vi "HFRR ADV v01.vi"() -> ()   [LabVIEW 2025] (continued)
            n2592 = Concatenate Strings(w3366, ".duf" ("Substring")) -> (w3363:string)
            n2593 = String To Path(string=w3363) -> (path=w3361:path)
            n2594 = call <vilib>:"Read Characters From File.vi"("file path (dialog if empty)"=w3361, "start of read offset (chars.:0)"=60 ("start of read offset (chars.: 0)")) -> ("character string"=→"String Control 4":string)  [unwired: 4 in, 3 out]
          }
        }
        n2595 = case shown="True" "OPEN 3" {
          frame False {
          }
          frame True {
            (unwired) 0  # existing file
            w3387 = "Choose a datalog file to open"  # prompt
            n2596 = local write "OPEN 3"(FALSE ("OPEN 1")) -> ()
            n2597 = String To Path(string="C:\\LAB-IQ\\Data\\") -> (path=w3372:path)
            n2598 = File Dialog(6:"*.dgf" ("pattern"), 7:w3387, 11:w3372) -> (0:w3370:errorcluster, 3:w3378:path)  [unwired: 4 in, 2 out]
            n2599 = Unbundle(w3370) -> ()  [unwired: 3 out]
            n2600 = Strip Path(path=w3378) -> (name=w3376:string)  [unwired: 1 out]
            n2601 = Path To String(path=w3378) -> (string=w3373:string)
            "string1 3" <- w3373
            n2602 = Match Pattern(string=w3376, regular expression=".dgf") -> (before substring=→"String Control 5":string)  [unwired: 1 in, 3 out]
            n2603 = Match Pattern(string=w3373, regular expression=".dgf" ("substring (\"\")")) -> (before substring=w3383:string)  [unwired: 1 in, 3 out]
            n2604 = Concatenate Strings(w3383, ".duf" ("Substring")) -> (w3380:string)
            n2605 = String To Path(string=w3380) -> (path=w3384:path)
            n2606 = call <vilib>:"Read Characters From File.vi"("file path (dialog if empty)"=w3384, "start of read offset (chars.:0)"=60 ("start of read offset (chars.: 0)")) -> ("character string"=→"String Control 6":string)  [unwired: 4 in, 3 out]
          }
        }
        n2607 = case shown="True" "OPEN 4" {
          frame False {
          }
          frame True {
            (unwired) 0  # existing file
            w3405 = "Choose a datalog file to open"  # prompt
            n2608 = local write "OPEN 4"(FALSE ("OPEN 1")) -> ()
            n2609 = String To Path(string="C:\\LAB-IQ\\Data\\") -> (path=w3390:path)
            n2610 = File Dialog(6:"*.dgf" ("pattern"), 7:w3405, 11:w3390) -> (0:w3388:errorcluster, 3:w3396:path)  [unwired: 4 in, 2 out]
            n2611 = Unbundle(w3388) -> ()  [unwired: 3 out]
            n2612 = Strip Path(path=w3396) -> (name=w3394:string)  [unwired: 1 out]
            n2613 = Path To String(path=w3396) -> (string=w3391:string)
            "string1 4" <- w3391
            n2614 = Match Pattern(string=w3394, regular expression=".dgf") -> (before substring=→"String Control 7":string)  [unwired: 1 in, 3 out]
            n2615 = Match Pattern(string=w3391, regular expression=".dgf" ("substring (\"\")")) -> (before substring=w3401:string)  [unwired: 1 in, 3 out]
            n2616 = Concatenate Strings(w3401, ".duf" ("Substring")) -> (w3398:string)
            n2617 = String To Path(string=w3398) -> (path=w3402:path)
            n2618 = call <vilib>:"Read Characters From File.vi"("file path (dialog if empty)"=w3402, "start of read offset (chars.:0)"=60 ("start of read offset (chars.: 0)")) -> ("character string"=→"String Control 8":string)  [unwired: 4 in, 3 out]
          }
        }
      }
      frame "About" {
        # "Elapsed time\ncof\nstroke\nmean pos\nTemp\nHumidity"
        n2619 = disable-structure shown="Disabled" {
          frame Disabled {
            n2620 = case shown="True" "Export" {
              frame False {
              }
              frame True {
                w3427 = "                                      " ("string")
                w3429 = "\r"
                (unwired) i16 6 ("width (-)")
                w3506 = "\r"
                w3438 = "\r"
                n2621 = local write "Export"(FALSE ("Export")) -> ()
                n2622 = local read "String 29"() -> (w3475:string)
                n2623 = local read "String 34"() -> (w3463:string)
                n2624 = local read "String 35"() -> (w3458:string)
                n2625 = local read "String 37"() -> (w3454:string)
                n2626 = local read "String 36"() -> (w3451:string)
                n2627 = local read "String 38"() -> (w3448:string)
                n2628 = local read "String 39"() -> (w3445:string)
                n2629 = Match Pattern(string=w3475, regular expression=".dwm") -> (before substring=w3471:string)  [unwired: 1 in, 3 out]
                "before substring" <- w3471
                n2630 = local read "S 38"() -> (w3466:string)
                n2631 = local read "S 39"() -> (w3459:string)
                n2632 = local read "Temperature before test 2"() -> (w3495:dbl)
                n2633 = local read "Temperature after test 2"() -> (w3500:dbl)
                n2634 = local read "Humidity before test 2"() -> (w3481:dbl)
                n2635 = local read "Humidity after test 2"() -> (w3496:dbl)
                n2636 = local read "MWSD 2"() -> (w3492:dbl)
                n2637 = local read "WS1.4 2"() -> (w3508:dbl)
                n2638 = local read "HCF 2"() -> (w3504:dbl)
                n2639 = local read "AVP 2"() -> (w3493:dbl)
                n2640 = Concatenate Strings("1," ("string"), w3466) -> (w3465:string)
                n2641 = Concatenate Strings("2," ("string"), w3463) -> (w3462:string)
                n2642 = Concatenate Strings("3," ("string"), w3459) -> (w3461:string)
                n2643 = Concatenate Strings("4," ("string"), w3458) -> (w3457:string)
                n2644 = Concatenate Strings("5," ("string"), w3454) -> (w3455:string)
                n2645 = Concatenate Strings("6," ("string"), w3451) -> (w3452:string)
                n2646 = Concatenate Strings("7," ("string"), w3448) -> (w3449:string)
                n2647 = Concatenate Strings("8," ("string"), w3445) -> (w3446:string)
                n2648 = local read "Sample ID"() -> (w3513:string)
                n2649 = case shown="\"xlx\"" "Select File Type" {
                  tunnel: w3471 -> [w3516 w3518 w3520]
                  tunnel: [w3514 w3519 w3521] -> w3470
                  frame "xlx" {
                    n2650 = Concatenate Strings(w3516, ".xls" ("string")) -> (w3514:string)
                  }
                  frame "csv" {
                    n2651 = Concatenate Strings(w3518, ".csv" ("string")) -> (w3519:string)
                  }
                  frame "txt" {
                    n2652 = Concatenate Strings(w3520, ".txt" ("string")) -> (w3521:string)
                  }
                }
                n2653 = local read "Test Date"() -> (w3512:string)
                n2654 = local read "String 45"() -> (w3426:string)
                n2655 = local read "String 31"() -> (w3511:string)
                n2656 = local read "String 32"() -> (w3510:string)
                n2657 = local read "TITTLE"() -> (w3434:string)
                n2658 = Number To Fractional String(number=w3481, width (-)=i16 6, precision (6)=i16 2) -> (F-format string=w3480:string)  [unwired: 1 in]
                n2659 = Number To Fractional String(number=w3495, width (-)=i16 6, precision (6)=i16 2) -> (F-format string=w3501:string)  [unwired: 1 in]
                n2660 = Number To Fractional String(number=w3496, width (-)=i16 6, precision (6)=i16 2) -> (F-format string=w3494:string)  [unwired: 1 in]
                n2661 = Number To Fractional String(number=w3500, width (-)=i16 6, precision (6)=i16 2) -> (F-format string=w3499:string)  [unwired: 1 in]
                n2662 = Number To Fractional String(number=w3492, width (-)=i16 6, precision (6)=i16 2) -> (F-format string=w3490:string)  [unwired: 1 in]
                n2663 = Number To Fractional String(number=w3493, width (-)=i16 6, precision (6)=i16 2) -> (F-format string=w3491:string)  [unwired: 1 in]
                n2664 = Number To Fractional String(number=w3504, width (-)=i16 6, precision (6)=i16 2) -> (F-format string=w3505:string)  [unwired: 1 in]
                n2665 = Number To Fractional String(number=w3508, precision (6)=i16 2) -> (F-format string=w3509:string)  [unwired: 2 in]
                n2666 = local read "s.NO"() -> (w3428:string)
                n2667 = Concatenate Strings("=" ("string"), w3434) -> (w3433:string)
                n2668 = Concatenate Strings("S.No," ("string"), "                                       Parameters" ("string")) -> (w3439:string)
                n2669 = Concatenate Strings(w3506, w3465, w3480, w3506, w3462, w3501, w3506, w3461, w3494, w3506, w3457, w3499, w3506, w3455, w3490, w3506, w3452, w3491, w3506, w3449, w3505, w3506, w3446, w3509) -> (w3468:string)
                n2670 = Concatenate Strings(w3438, "," ("string"), w3426, w3428, w3427, w3510, w3513, w3427, w3511, w3512, w3438) -> (w3436:string)
                n2671 = local read "Tested by"() -> (w3442:string)
                n2672 = local read "String 33"() -> (w3443:string)
                n2673 = Concatenate Strings("," ("string"), "                                                                             " ("string")) -> (w3431:string)
                n2674 = Concatenate Strings(w3433, w3429, w3436, w3429, w3439, w3468, w3429, w3431, w3443, w3442) -> (→"export":string)
                n2675 = String To Path(string=w3470) -> (path=w3477:path)
                n2676 = local read "export"() -> (w3472:string)
                n2677 = call <vilib>:"Write Characters To File.vi"("append to file? (new file:F)"=FALSE, "character string"=w3472, "file path (dialog if empty)"=w3477) -> ()  [unwired: 2 in, 1 out]
              }
            }
          }
          frame Enabled {
          }
        }
        n2678 = case shown="True" "OK Button 17" {
          frame False {
          }
          frame True {
            (unwired) 0  # existing file
            w3730 = "Choose a datalog file to open"  # prompt
            n2679 = local write "OK Button 17"(FALSE ("OK Button 17")) -> ()
            n2680 = local read "String"() -> (w3725:string)
            n2681 = String To Path(string=w3725) -> (path=w3726:path)
            n2682 = File Dialog(6:"*.duf" ("pattern"), 7:w3730, 11:w3726) -> (0:w3717:errorcluster, 3:w3736:path)  [unwired: 4 in, 2 out]
            n2683 = Unbundle(w3717) -> ()  [unwired: 3 out]
            n2684 = Open/Create/Replace File "Open File"(file path (use dialog)=w3736) -> (refnum out=w3728:refnum<file>)  [unwired: 5 in, 2 out]
            n2685 = Strip Path(path=w3736) -> (name=w3734:string)  [unwired: 1 out]
            n2686 = Path To String(path=w3736) -> (string=w3719:string)
            n2687 = while {
              tunnel: w3728 -> [w3740]
              i -> [w3737]
              stop <- w3738 continue-if-true
              (unwired) TRUE ("line mode (F)")
              n2688 = Read from Text File "Read File"(file (use dialog)=w3740) -> (text=w3739:string)  [unwired: 3 in, 3 out]
              n2689 = local write "Numeric 16"(w3737) -> ()
              n2690 = String Length(string=w3739) -> (length=w3742:i32)
              n2691 = Greater?(x=w3742, y=1) -> (0:w3738:bool)
            }
            n2692 = local write "String 29"(w3719) -> ()
            n2693 = Search and Replace String(input string=w3719, search string=".duf", replace string=".dgf" ("replace string (\"\")")) -> (result string=→"String Indicator 4":string)  [unwired: 5 in, 3 out]
            n2694 = Match Pattern(string=w3734, regular expression=".dwm") -> (before substring=w3718:string)  [unwired: 1 in, 3 out]
            "String Indicator" <- w3718
            n2695 = Match Pattern(string=w3719, regular expression=".dwm" ("substring (\"\")")) -> (before substring=w3720:string)  [unwired: 1 in, 3 out]
            "String Indicator 3" <- w3720
            n2696 = local write "TITTLE 2"(w3718) -> ()
            n2697 = String To Path(string=w3720) -> (path=w3727:path)
            "path" <- w3727
            n2698 = call <vilib>:"Read Characters From File.vi"("file path (dialog if empty)"=w3727, "start of read offset (chars.:0)"=60 ("start of read offset (chars.: 0)")) -> ("character string"=→"String Indicator 2":string)  [unwired: 4 in, 3 out]
          }
        }
        n2699 = call <vilib>:"Query Available Printers.vi"() -> ("system configured printers"=w3419:string[])  [unwired: 9 in, 2 out]
        "System Configured Printers 2" <- w3419
        n2700 = local read "OK Button 16"() -> (w3416:bool)
        n2701 = case shown="True" "OK Button 16" {
          frame False {
          }
          frame True {
            n2702 = stacked-sequence {
              frame #0 {
                n2703 = local read "Numeric 16"() -> (w3744:i32)
                n2704 = local write "Numeric 10"(w3744) -> ()
              }
              frame #1 {
                n2705 = local read "S.NO"() -> (→"s.NO":string)
                n2706 = local read "String 29"() -> (w3748:string)
                n2707 = String To Path(string=w3748) -> (path=w3747:path)
                n2708 = Open/Create/Replace File "Open File"(file path (use dialog)=w3747) -> (refnum out=w3749:refnum<file>)  [unwired: 5 in, 2 out]
                n2709 = for {
                  N: 16 -> [_]
                  tunnel: w3749 -> [w3756]
                  i -> [w3752]
                  (unwired) TRUE ("line mode (F)")
                  n2710 = Read from Text File "Read File"(file (use dialog)=w3756) -> (text=w3750:string)  [unwired: 3 in, 3 out]
                  n2711 = Match Pattern(string=w3750, regular expression="(") -> (after substring=w3755:string)  [unwired: 1 in, 3 out]
                  n2712 = Match Pattern(string=w3755, regular expression=")") -> (before substring=w3751:string)  [unwired: 1 in, 3 out]
                  n2713 = case shown="1" w3752 {
                    tunnel: w3751 -> [w3757 w3758 _ _ w3759 w3760 w3761 w3763 w3765 w3767 w3769 w3771 w3773 w3775 _]
                    tunnel: w3750 -> [_ _ _ _ _ _ _ _ _ _ _ _ _ _ _]
                    frame 0 {
                      "TITTLE" <- w3757
                    }
                    frame 1 {
                      "Sample ID" <- w3758
                    }
                    frame 2 {
                    }
                    frame 3 {
                    }
                    frame 4 {
                      "Test Date" <- w3759
                    }
                    frame 5 {
                      "Tested by" <- w3760
                    }
                    frame 6 {
                      n2714 = Fract/Exp String To Number(string=w3761) -> (number=→"Humidity before test 2":dbl)  [unwired: 3 in, 1 out]
                    }
                    frame 7 {
                      n2715 = Fract/Exp String To Number(string=w3763) -> (number=→"Temperature before test 2":dbl)  [unwired: 3 in, 1 out]
                    }
                    frame 8 {
                      n2716 = Fract/Exp String To Number(string=w3765) -> (number=→"Humidity after test 2":dbl)  [unwired: 3 in, 1 out]
                    }
                    frame 9 {
                      n2717 = Fract/Exp String To Number(string=w3767) -> (number=→"Temperature after test 2":dbl)  [unwired: 3 in, 1 out]
                    }
                    frame 10 {
                      n2718 = Fract/Exp String To Number(string=w3769) -> (number=→"MWSD 2":dbl)  [unwired: 3 in, 1 out]
                    }
                    frame 11 {
                      n2719 = Fract/Exp String To Number(string=w3771) -> (number=→"AVP 2":dbl)  [unwired: 3 in, 1 out]
                    }
                    frame 12 {
                      n2720 = Fract/Exp String To Number(string=w3773) -> (number=→"HCF 2":dbl)  [unwired: 3 in, 1 out]
                    }
                    frame 13 {
                      n2721 = Fract/Exp String To Number(string=w3775) -> (number=→"WS1.4 2":dbl)  [unwired: 3 in, 1 out]
                    }
                    frame 14, Default {
                    }
                  }
                }
              }
              frame #2 {
              }
            }
            n2722 = local write "OK Button 16"(FALSE ("OK Button 13")) -> ()
          }
        }
        n2723 = Index Array(array=w3419, index="Select Printer 3") -> (element=w3421:string)
        "Selected Printer" <- w3421
        n2724 = case shown="True" w3416 {
          frame False {
          }
          frame True {
            n2725 = flat-sequence {
              frame #0 {
              }
              frame #1 {
                n2726 = Wait (ms)(milliseconds to wait=u32 100) -> ()  [unwired: 1 out]
              }
              frame #2 {
                n2727 = local write "OK Button 16"(FALSE ("Print 3")) -> ()
              }
            }
          }
        }
        n2728 = case shown="True" "Print" {
          tunnel: w3421 -> [_ w3713]
          frame False {
          }
          frame True {
            (unwired) i16 6 ("width (-)")
            (unwired) "TESTED BY : "
            (unwired) "TESTED DATE :"
            (unwired) "SAMPLE ID : "
            (unwired) "SAMPLE DESIGN : "
            w3671 = "\r"
            w3688 = "\r"
            # "add image"
            n2729 = local read "Sample ID"() -> (w3661:string)
            n2730 = local read "Tested by"() -> (w3664:string)
            n2731 = local read "String 34"() -> (w3651:string)
            n2732 = local read "String 45"() -> (w3631:string)
            n2733 = local read "String 35"() -> (w3646:string)
            n2734 = local read "String 37"() -> (w3644:string)
            n2735 = local read "String 32"() -> (w3666:string)
            n2736 = local read "String 36"() -> (w3641:string)
            n2737 = local read "String 31"() -> (w3665:string)
            n2738 = local read "Test Date"() -> (w3662:string)
            n2739 = local read "String 33"() -> (w3667:string)
            n2740 = local read "String 38"() -> (w3637:string)
            n2741 = local read "String 39"() -> (w3634:string)
            n2742 = local write "Print"(FALSE ("Print FF")) -> ()
            n2743 = local read "S 39"() -> (w3649:string)
            n2744 = local read "S 38"() -> (w3656:string)
            n2745 = local read "Temperature before test 2"() -> (w3687:dbl)
            n2746 = local read "Temperature after test 2"() -> (w3677:dbl)
            n2747 = local read "Humidity before test 2"() -> (w3702:dbl)
            n2748 = local read "Humidity after test 2"() -> (w3686:dbl)
            n2749 = local read "MWSD 2"() -> (w3691:dbl)
            n2750 = local read "WS1.4 2"() -> (w3669:dbl)
            n2751 = Concatenate Strings("2)" ("string"), w3651) -> (w3652:string)
            n2752 = Concatenate Strings("3)" ("string"), w3649) -> (w3650:string)
            n2753 = Concatenate Strings("1)" ("string"), w3656) -> (w3655:string)
            n2754 = Concatenate Strings("4)" ("string"), w3646) -> (w3647:string)
            n2755 = Concatenate Strings("5)" ("string"), w3644) -> (w3643:string)
            n2756 = Concatenate Strings("6)" ("string"), w3641) -> (w3640:string)
            n2757 = Concatenate Strings("7)" ("string"), w3637) -> (w3638:string)
            n2758 = Concatenate Strings("8)" ("string"), w3634) -> (w3635:string)
            n2759 = local read "HCF 2"() -> (w3673:dbl)
            n2760 = local read "AVP 2"() -> (w3690:dbl)
            n2761 = local read "s.NO"() -> (w3632:string)
            n2762 = call <vilib>:"New Report.vi"("report type"=enum16{"Standard Report", "HTML"}."Standard Report") -> ("report out"=w3711:refnum<class "NI_report.lvclass">, "error out"=w3710:errorcluster)  [unwired: 13 in]
            n2763 = local read "TITTLE"() -> (w3663:string)
            n2764 = Concatenate Strings(w3688, w3631, w3632, w3688, w3666, w3661, w3688, w3665, w3662, w3688, w3667, w3664, w3688) -> (w3681:string)
            "test by" <- w3681
            n2765 = Number To Fractional String(number=w3687, width (-)=i16 6, precision (6)=i16 2) -> (F-format string=w3676:string)  [unwired: 1 in]
            n2766 = Number To Fractional String(number=w3686, width (-)=i16 6, precision (6)=i16 2) -> (F-format string=w3689:string)  [unwired: 1 in]
            n2767 = Number To Fractional String(number=w3702, width (-)=i16 6, precision (6)=i16 2) -> (F-format string=w3707:string)  [unwired: 1 in]
            n2768 = Number To Fractional String(number=w3691, width (-)=i16 6, precision (6)=i16 2) -> (F-format string=w3693:string)  [unwired: 1 in]
            n2769 = Number To Fractional String(number=w3677, width (-)=i16 6, precision (6)=i16 2) -> (F-format string=w3678:string)  [unwired: 1 in]
            n2770 = Number To Fractional String(number=w3690, width (-)=i16 6, precision (6)=i16 2) -> (F-format string=w3692:string)  [unwired: 1 in]
            n2771 = Number To Fractional String(number=w3673, width (-)=i16 6, precision (6)=i16 2) -> (F-format string=w3672:string)  [unwired: 1 in]
            n2772 = Number To Fractional String(number=w3669, precision (6)=i16 2) -> (F-format string=w3668:string)  [unwired: 2 in]
            n2773 = call-dynamic "Set Report Header Text.vi"("report in"=w3711, "center header text"=w3663, "error in (no error)"=w3710) -> ("report out"=w3682:refnum<class "NI_report.lvclass">, "error out"=w3683:errorcluster)  [unwired: 11 in]
            n2774 = Concatenate Strings(w3671, w3655, w3707, w3671, w3652, w3676, w3671, w3650, w3689, w3671, w3647, w3678, w3671, w3643, w3693, w3671, w3640, w3692, w3671, w3638, w3672, w3671, w3635, w3668) -> (w3659:string)
            "export 2" <- w3659
            n2775 = call-poly <vilib>:"Append Report Text.vi"("report in"=w3682, "text"=w3681, "error in (no error)"=w3683) -> ("report out"=w3685:refnum<class "NI_report.lvclass">, "error out"=w3684:errorcluster)  [unwired: 9 in, 2 out]
            n2776 = local read "test by"() -> (w3658:string)
            n2777 = local read "TITTLE"() -> (w3660:string)
            n2778 = call-poly <vilib>:"Append Report Text.vi"("report in"=w3685, "error in (no error)"=w3684) -> ("report out"=w3706:refnum<class "NI_report.lvclass">, "error out"=w3704:errorcluster)  [unwired: 10 in, 2 out]
            n2779 = Concatenate Strings(w3660, w3659, w3658) -> (→"output":string)
            n2780 = call-poly <vilib>:"Append Report Text.vi"("report in"=w3706, "text"=w3659, "error in (no error)"=w3704) -> ("report out"=w3705:refnum<class "NI_report.lvclass">, "error out"=w3703:errorcluster)  [unwired: 9 in, 2 out]
            n2781 = call-dynamic "Print Report.vi"("report in"=w3705, "printer name (default)"=w3713, "error in (no error)"=w3703) -> ("report out"=w3715:refnum<class "NI_report.lvclass">, "error out"=w3716:errorcluster)  [unwired: 11 in]
            n2782 = call-dynamic "Dispose Report.vi"("report in"=w3715, "error in (no error)"=w3716) -> ()  [unwired: 13 in, 1 out]
          }
        }
        n2783 = case shown="True" "Print 2" {
          frame False {
          }
          frame True {
            n2784 = flat-sequence {
              frame #0 {
                n2785 = local read "s.NO"() -> (→"s.NO 2":string)
                n2786 = Wait (ms)(milliseconds to wait=u32 20) -> ()  [unwired: 1 out]
                n2787 = local read "Sample ID  3"() -> (→"Sample ID  6":string)
                n2788 = local read "Sample ID  4"() -> (→"Sample ID  7":string)
                n2789 = local read "Sample ID"() -> (→"Sample ID  2":string)
                n2790 = local read "Tested by"() -> (→"Tested by 2":string)
                n2791 = local read "Test Date"() -> (→"Test Date 2":string)
                n2792 = local read "Humidity after test 3"() -> (→"Humidity after test 4":dbl)
                n2793 = local read "Ref A Test Date :"() -> (→"TITTLE 4":string)
                n2794 = local read "Temperature before test 3"() -> (w3538:dbl)
                n2795 = local read "Temperature before test 3"() -> (→"Temperature after test 5":dbl)
                n2796 = local read "Temperature after test 3"() -> (→"Temperature after test 4":dbl)
                n2797 = local read "Humidity before test 3"() -> (→"Humidity before test 4":dbl)
                n2798 = local write "Temperature before test 3"(w3538) -> ()
                n2799 = local read "image data"() -> (w3529:T13)
                n2800 = String To Path(string="C:\\LAB-IQ\\im\\Temp_resized.jpg") -> (path=w3530:path)
                "path 2" <- w3530
                n2801 = call <vilib>:"Write JPEG File.vi"("image data"=w3529, "path to JPEG file"=w3530) -> ()  [unwired: 8 in, 2 out]
                "Ref A Test Date :" <- "Ref A Test Date :"
                "Ref B Test Date :" <- "Ref B Test Date :"
                "Ref B Scar Value :" <- "Ref B Scar Value :"
                "Ref A Scar Value :" <- "Ref A Scar Value :"
              }
              frame #1 {
                (unwired) HTML_Report_Image_Alignment."MIDDLE" ("alignment (default)")
                w3566 = u16 0 items=["portrait", "landscape"] ("orientation (portrait)")
                (unwired) HTML_Report_Image_Alignment."ABSMIDDLE" ("alignment (default)")
                (unwired) "TESTED BY : "
                (unwired) "TESTED DATE :"
                (unwired) "SAMPLE ID : "
                (unwired) "SAMPLE DESIGN : "
                w3599 = "\r"
                # "add image"
                n2802 = Wait (ms)(milliseconds to wait=u32 20) -> ()  [unwired: 1 out]
                n2803 = local read "Sample ID  2"() -> (w3592:string)
                n2804 = local read "Wear Scar X"() -> (w3564:dbl)
                "Length ( microns ) 2" <- w3564
                n2805 = local read "Wear Scar Y"() -> (w3563:dbl)
                "Wear Scar Y ( microns ) :" <- w3563
                n2806 = local read "Test Date 2"() -> (w3593:string)
                n2807 = local read "Tested by 2"() -> (w3594:string)
                n2808 = local read "String 46"() -> (w3590:string)
                n2809 = local read "String 48"() -> (w3596:string)
                n2810 = local read "String 47"() -> (w3595:string)
                n2811 = local read "String 49"() -> (w3597:string)
                n2812 = local read "String 10"() -> (w3550:string)
                n2813 = local read "s.NO 2"() -> (w3591:string)
                n2814 = Add(x=w3564, y=w3563) -> (x+y=w3562:dbl)
                n2815 = call <vilib>:"New Report.vi"("report type"=enum16{"Standard Report", "HTML"}."HTML") -> ("report out"=w3570:refnum<class "NI_report.lvclass">, "error out"=w3568:errorcluster)  [unwired: 13 in]
                n2816 = Concatenate Strings(w3599, w3590, w3591, w3599, w3596, w3592, w3599, w3595, w3593, w3599, w3597, w3594, w3599) -> (→"test by 2":string)
                n2817 = Concatenate Strings("C:\\LAB-IQ\\Data\\" ("string"), w3550, ".jpg" ("string")) -> ()  [unwired: 1 out]
                n2818 = Divide(x=w3562, y=2.0) -> (x/y=→"Mean Wear ( microns) :":dbl)
                n2819 = call-dynamic "Set Report Orientation.vi"("report in"=w3570, "orientation (portrait)"=w3566, "error in (no error)"=w3568) -> ("report out"=w3569:refnum<class "NI_report.lvclass">, "error out"=w3567:errorcluster)  [unwired: 11 in]
                n2820 = for {
                  N: 5 -> [_]
                  tunnel: w3569 -> [w3620]
                  tunnel: [w3619] -> w3548
                  tunnel: w3567 -> [w3618]
                  tunnel: [w3617] -> w3547
                  n2821 = call-dynamic "Set Report Tab Width.vi"("report in"=w3620, "error in (no error)"=w3618) -> ("report out"=w3619:refnum<class "NI_report.lvclass">, "error out"=w3617:errorcluster)  [unwired: 12 in]
                }
                n2822 = local read "TITTLE"() -> (w3565:string)
                n2823 = call-dynamic "Set Report Header Text.vi"("report in"=w3548, "center header text"=w3565, "error in (no error)"=w3547) -> ("report out"=w3586:refnum<class "NI_report.lvclass">, "error out"=w3585:errorcluster)  [unwired: 11 in]
                n2824 = for {
                  N: 1 -> [_]
                  tunnel: [w3624] -> w3572
                  tunnel: [w3623] -> w3571
                  tunnel: w3586 -> [w3622]
                  tunnel: w3585 -> [w3621]
                  n2825 = call-dynamic "New Report Line.vi"("report in"=w3622, "error in (no error)"=w3621) -> ("report out"=w3624:refnum<class "NI_report.lvclass">, "error out"=w3623:errorcluster)  [unwired: 12 in]
                }
                n2826 = for {
                  N: 2 -> [_]
                  tunnel: [w3616] -> w3578
                  tunnel: [w3615] -> w3577
                  tunnel: w3572 -> [w3614]
                  tunnel: w3571 -> [w3613]
                  n2827 = call-dynamic "New Report Line.vi"("report in"=w3614, "error in (no error)"=w3613) -> ("report out"=w3616:refnum<class "NI_report.lvclass">, "error out"=w3615:errorcluster)  [unwired: 12 in]
                }
                n2828 = for {
                  N: 25 -> [_]
                  tunnel: w3578 -> [w3612]
                  tunnel: w3577 -> [w3610]
                  tunnel: [w3611] -> w3581
                  tunnel: [w3609] -> w3580
                  n2829 = call-dynamic "Set Report Tab Width.vi"("report in"=w3612, "error in (no error)"=w3610) -> ("report out"=w3611:refnum<class "NI_report.lvclass">, "error out"=w3609:errorcluster)  [unwired: 12 in]
                }
                n2830 = control-ref of="Tab Control 9"() -> (w3576:refnum<vi>)
                n2831 = call-dynamic "Append Control Image to Report.vi"("report in"=w3581, "alignment (default)"=HTML_Report_Image_Alignment."ABSMIDDLE", "ctrl reference"=w3576, "error in (no error)"=w3580) -> ("report out"=w3575:refnum<class "NI_report.lvclass">, "error out"=w3574:errorcluster)  [unwired: 8 in, 2 out]
                n2832 = for {
                  N: 3 -> [_]
                  tunnel: [w3608] -> w3559
                  tunnel: [w3607] -> w3558
                  tunnel: w3575 -> [w3606]
                  tunnel: w3574 -> [w3605]
                  n2833 = call-dynamic "New Report Line.vi"("report in"=w3606, "error in (no error)"=w3605) -> ("report out"=w3608:refnum<class "NI_report.lvclass">, "error out"=w3607:errorcluster)  [unwired: 12 in]
                }
                n2834 = for {
                  N: 100 -> [_]
                  tunnel: w3559 -> [w3604]
                  tunnel: w3558 -> [w3602]
                  tunnel: [w3603] -> w3555
                  tunnel: [w3601] -> w3553
                  n2835 = call-dynamic "Set Report Tab Width.vi"("report in"=w3604, "error in (no error)"=w3602) -> ("report out"=w3603:refnum<class "NI_report.lvclass">, "error out"=w3601:errorcluster)  [unwired: 12 in]
                }
                n2836 = String To Path(string="C:\\LAB-IQ\\im\\Temp_resized.jpg") -> (path=w3545:path)
                n2837 = call-poly <vilib>:"Append Image to Report.vi"("report in"=w3555, "path or URL of image"=w3545, "error in (no error)"=w3553) -> ("report out"=w3554:refnum<class "NI_report.lvclass">, "error out"=w3552:errorcluster)  [unwired: 9 in, 2 out]
                n2838 = call-poly <vilib>:"Open HTML Report in Browser.vi"("report in"=w3554, "error in (no error)"=w3552) -> ("report out"=w3589:refnum<class "NI_report.lvclass">, "error out"=w3588:errorcluster)  [unwired: 11 in, 1 out]
                n2839 = call-dynamic "Dispose Report.vi"("report in"=w3589, "error in (no error)"=w3588) -> ()  [unwired: 13 in, 1 out]
              }
              frame #2 {
              }
              frame #3 {
                n2840 = disable-structure shown="Disabled" {
                  frame Disabled {
                    n2841 = local read "String 10"() -> (w3629:string)
                    n2842 = Concatenate Strings("C:\\LAB-IQ-NXT\\Data\\" ("string"), w3629, ".jpg" ("string")) -> (w3627:string)
                    n2843 = String To Path(string=w3627) -> (path=w3626:path)
                    n2844 = Delete(path (use dialog)=w3626) -> ()  [unwired: 4 in, 3 out]
                  }
                  frame Enabled {
                  }
                }
                n2845 = local write "Print 2"(FALSE ("Print")) -> ()
              }
            }
          }
        }
      }
    }
    n2846 = property on="SetTemp" class="DigNum (strict)"("Disabled"=w1582) -> ()  [unwired: 2 in, 2 out]
    n2847 = Multiply(x=w1571, y=w1573) -> (x*y=w1572:dbl)
    n2848 = local read "MWSD"() -> (w1570:dbl)
    n2849 = Add(x=w1572, y=w1570) -> (x+y=→"WS1.4":dbl)
    n2850 = Wait (ms)(milliseconds to wait=u32 50) -> ()  [unwired: 1 out]
    n2851 = Wait (ms)(milliseconds to wait=u32 50) -> ()  [unwired: 1 out]
    n2852 = local read "Quit"() -> (w1569:bool)
  }
  n2853 = VISA Close(VISA resource name=w50, error in (no error)=w49) -> (error out=w47:errorcluster)
  n2854 = call <vilib>:"Clear Errors.vi"("error in (no error)"=w47) -> ()  [unwired: 5 in, 2 out]
  n2855 = VISA Close(VISA resource name=w34, error in (no error)=w33) -> ()  [unwired: 1 out]
  n2856 = Or(x=w39, y=w38) -> (x .or. y?=w40:bool)
  n2857 = while {
    tunnel: [w3780] -> w44
    tunnel: [w3781] -> _
    i -> [w3781]
    stop <- w3780 stop-if-true
    # "PID LOGIC"
    n2858 = Wait (ms)(milliseconds to wait=u32 80) -> ()  [unwired: 1 out]
    n2859 = local read "Quit"() -> (w3780:bool)
    n2860 = local read "Due Com"() -> (w3778:string[])
    n2861 = Build Array (concatenate)(w3778, "") -> (→"Due Com":string[])
  }
  n2862 = Or(x=w36, y=w40) -> (x .or. y?=w46:bool)
  n2863 = control-ref of="new picture"() -> ()  [unwired: 1 out]
  n2864 = Or(x=w52, y=w46) -> (x .or. y?=w43:bool)
  n2865 = Or(x=w43, y=w44) -> (x .or. y?=w37:bool)
  n2866 = while {
    tunnel: [w3783] -> w51
    i -> [w3790]
    stop <- w3783 stop-if-true
    n2867 = local read "Quit"() -> (w3783:bool)
    n2868 = Equal To 0?(x=w3790) -> (x = 0?=w3788:bool)
    n2869 = call "Elapsed Time3"("Time Target (s)"=45.0, "Auto Reset"=TRUE) -> ("Time has Elapsed"=w3787:bool)  [unwired: 10 in, 7 out]
    n2870 = Wait (ms)(milliseconds to wait=u32 50) -> ()  [unwired: 1 out]
    n2871 = Or(x=w3787, y=w3788) -> (x .or. y?=w3789:bool)
    n2872 = case shown="True" w3789 {
      frame False {
      }
      frame True {
        n2873 = call <vilib>:"System Exec.vi"("run minimized? (F)"=TRUE, "error in (no error)"="error in (no error)", "command line"="powercfg.exe -change -monitor-timeout-ac 0") -> ("error out"=w3801:errorcluster)  [unwired: 5 in, 3 out]
        n2874 = call <vilib>:"System Exec.vi"("run minimized? (F)"=TRUE, "error in (no error)"=w3801, "command line"="powercfg.exe -change -disk-timeout-ac 0") -> ("error out"=w3800:errorcluster)  [unwired: 5 in, 3 out]
        n2875 = call <vilib>:"System Exec.vi"("run minimized? (F)"=TRUE, "error in (no error)"=w3800, "command line"="powercfg.exe -change -standby-timeout-ac 0") -> ("error out"=w3799:errorcluster)  [unwired: 5 in, 3 out]
        n2876 = call <vilib>:"System Exec.vi"("run minimized? (F)"=TRUE, "error in (no error)"=w3799, "command line"="powercfg.exe -change -hibernate-timeout-ac 0") -> ("error out"=w3798:errorcluster)  [unwired: 5 in, 3 out]
        n2877 = call <vilib>:"Simple Error Handler.vi"("error in (no error)"=w3798) -> ("error out"=w3804:errorcluster)  [unwired: 4 in, 4 out]
        n2878 = call <vilib>:"Clear Errors.vi"("error in (no error)"=w3804) -> ("error out"=→"error out":errorcluster)  [unwired: 5 in, 1 out]
      }
    }
  }
  n2879 = Compound Arithmetic op=OR(w54, w37, w51) -> (w53:bool)
  n2880 = flat-sequence {
    tunnel: w53 -> [_]
    tunnel: [w3806] -> w14
    tunnel: w14 -> [_]
    frame #0 {
      n2881 = call "CLOSE CONNECTION.vi"() -> ("error out"=w3806:errorcluster)  [unwired: 11 in]
    }
    frame #1 {
      n2882 = Quit LabVIEW(quit? (T)=TRUE) -> ()
      n2883 = local write "Quit"(FALSE ("EXIT")) -> ()
    }
  }
  n2884 = property on="Heater Button" class="Bool (strict)"("Visible"=TRUE) -> ()  [unwired: 2 in, 2 out]
  n2885 = disable-structure shown="Disabled" {
    disable-tunnel: _ -> [w3812 _]
    disable-tunnel: _ -> [w3809 _]
    disable-tunnel: _ -> [w3810 _]
    frame Disabled {
      n2886 = disable-structure shown="Disabled" {
        disable-tunnel: [w3819 _] -> w3811
        frame Disabled {
          n2887 = while {
            shift-right: [w3861] -> w3817
            shift-left: errorcluster {"status"=TRUE, "code"=0, "source"="Init"} ("error out") -> [w3826]
            shift-right: [w3860] -> w3816
            shift-left: _ -> [w3827]
            shift-right: [w3859] -> _
            shift-left: "" -> [w3858]
            tunnel: [w3820] -> w3819
            shift-right: ["Set Rh"] -> _
            shift-left: 0.0 ("Set Rh") -> [w3852]
            tunnel: [w3829] -> _
            i -> [w3829]
            stop <- w3820 stop-if-true
            n2888 = flat-sequence {
              tunnel: w3826 -> [w3864]
              tunnel: [w3864] -> w3825
              frame #0 {
                n2889 = Wait (ms)(milliseconds to wait=u32 200) -> ()  [unwired: 1 out]
              }
            }
            n2890 = local read "Com Port 3"() -> (w3828:refnum<visa-resource-name>)
            n2891 = local read "Humidity Str Rec"() -> (w3830:string)
            n2892 = Not Equal?(x="Set Rh", y=w3852) -> (x != y?=w3857:bool)
            n2893 = Number To Decimal String(number="Set Rh") -> (decimal integer string=w3855:string)  [unwired: 1 in]
            n2894 = Not Equal?(x=w3828, y=w3827) -> (x != y?=w3823:bool)
            n2895 = Concatenate Strings("#setPoint00" ("string"), w3855) -> (w3856:string)
            n2896 = case shown="False" w3857 {
              tunnel: w3856 -> [_ w3876]
              frame False {
                n2897 = local read "Humidity"() -> (w3873:bool)
                n2898 = case shown="True" w3873 {
                  frame False {
                    n2899 = local write "Humidity Str Send"("stop" ("Humidity Str Send")) -> ()
                  }
                  frame True {
                    n2900 = local write "Humidity Str Send"("start" ("Humidity Str Send")) -> ()
                  }
                }
              }
              frame True {
                n2901 = local write "Humidity Str Send"(w3876) -> ()
              }
            }
            n2902 = Or(x=w3823, y="Re-Initialise") -> (x .or. y?=w3822:bool)
            n2903 = String Subset(string=w3830, offset (0)=7) -> (substring=w3845:string)  [unwired: 1 in]
            n2904 = Match Pattern(string=w3830, regular expression="?") -> (offset past match=w3848:i32)  [unwired: 1 in, 3 out]
            n2905 = Match Pattern(string=w3830, regular expression="v") -> (offset past match=w3851:i32)  [unwired: 1 in, 3 out]
            n2906 = case shown="True" w3822 {
              tunnel: w3825 -> [w3862 _]
              tunnel: [w3862 errorcluster {"status"=TRUE, "code"=0, "source"="Init"} ("error out")] -> w3824
              frame False {
              }
              frame True {
              }
            }
            n2907 = Equal?(x=w3848, y=-1) -> (x = y?=w3832:bool)
            n2908 = Match Pattern(string=w3845, regular expression="g") -> (after substring=w3846:string, offset past match=w3837:i32)  [unwired: 1 in, 2 out]
            n2909 = Match Pattern(string=w3845, regular expression="y") -> (after substring=w3844:string, offset past match=w3838:i32)  [unwired: 1 in, 2 out]
            n2910 = Greater?(x=w3838, y=w3837) -> (0:w3843:bool)
            n2911 = Greater Or Equal To 0?(x=w3838) -> (x >= 0?=w3835:bool)
            n2912 = Greater Or Equal To 0?(x=w3837) -> (x >= 0?=w3836:bool)
            n2913 = Or(x=w3835, y=w3836) -> (x .or. y?=w3834:bool)
            n2914 = Greater Or Equal To 0?(x=w3851) -> (x >= 0?=w3833:bool)
            n2915 = Select(t=w3844, s=w3843, f=w3846) -> (s? t:f=w3839:string)
            n2916 = case shown="Error" w3824 {
              selector: w3824 -> [w3889 w3935]
              tunnel: [w3887 w3928] -> w3861
              tunnel: w3827 -> [w3890 w3934]
              tunnel: [w3888 w3937] -> w3860
              tunnel: w3858 -> [w3877 w3936]
              tunnel: [w3884 w3936] -> w3859
              frame No Error {
                n2917 = call "Elapsed Time7"() -> ("Time has Elapsed"=w3883:bool)  [unwired: 12 in, 7 out]
                n2918 = Not Equal?(x="Humidity Str Send", y=w3877) -> (x != y?=w3879:bool)
                n2919 = Or(x=w3879, y=w3883) -> (x .or. y?=w3882:bool)
                n2920 = Select(t="Humidity Str Send", s=w3879, f="vals" ("regular expression")) -> (s? t:f=w3878:string)
                n2921 = Or(x=w3882, y="Send") -> (x .or. y?=w3886:bool)
                n2922 = case shown="True" w3886 {
                  tunnel: [w3893 w3898] -> w3887
                  tunnel: w3890 -> [w3892 w3906]
                  tunnel: w3889 -> [w3893 w3905]
                  tunnel: [w3892 w3899] -> w3888
                  tunnel: w3878 -> [_ w3904]
                  tunnel: [w3891 w3895] -> w3884
                  tunnel: "Humidity Str Send" -> [_ w3896]
                  tunnel: w3879 -> [_ w3897]
                  tunnel: w3877 -> [w3891 w3894]
                  frame False {
                  }
                  frame True {
                    n2923 = flat-sequence {
                      tunnel: w3906 -> [w3914]
                      tunnel: w3905 -> [w3913]
                      tunnel: w3904 -> [w3910]
                      tunnel: [w3912] -> w3903
                      tunnel: [w3911] -> w3902
                      tunnel: w3903 -> [w3917]
                      tunnel: w3902 -> [w3916]
                      tunnel: [w3917] -> w3901
                      tunnel: [w3916] -> w3900
                      tunnel: w3901 -> [w3924]
                      tunnel: w3900 -> [w3923]
                      tunnel: [w3922] -> w3899
                      tunnel: [w3921] -> w3898
                      frame #0 {
                        n2924 = local write "Ser Led"(TRUE ("Boolean 4")) -> ()
                        n2925 = Concatenate Strings(w3910, "\r") -> (w3909:string)
                        n2926 = VISA Write(VISA resource name=w3914, write buffer=w3909, error in (no error)=w3913) -> (VISA resource name out=w3912:refnum<visa-resource-name>, error out=w3911:errorcluster)  [unwired: 1 out]
                      }
                      frame #1 {
                        n2927 = Wait (ms)(milliseconds to wait="wait") -> ()  [unwired: 1 out]
                      }
                      frame #2 {
                        w3919 = FALSE ("Send")
                        n2928 = property class="Instr"(reference=w3924, error in=w3923) -> (reference out=w3925:refnum<visa-resource-name>, error out=w3926:errorcluster, "Serial Settings:Number of Bytes at Serial Port"=w3918:u32)
                        "Humidity 2" <- w3918
                        n2929 = local write "Send"(w3919) -> ()
                        n2930 = local write "Ser Led"(w3919) -> ()
                        n2931 = VISA Read(VISA resource name=w3925, byte count=w3918, error in (no error)=w3926) -> (VISA resource name out=w3922:refnum<visa-resource-name>, read buffer=→"Humidity Str Rec":string, error out=w3921:errorcluster)  [unwired: 1 out]
                      }
                    }
                    n2932 = Select(t=w3896, s=w3897, f=w3894) -> (s? t:f=w3895:string)
                  }
                }
              }
              frame Error {
                w3942 = u16 0 items=["None"=0, "XON/XOFF"=1, "RTS/CTS"=2, "DTR/DSR"=4] ("flow control")
                w3938 = u16 0 items=["None", "Odd", "Even", "Mark", "Space"] ("parity")
                w3941 = u16 10 items=["1.0"=10, "1.5"=15, "2.0"=20] ("stop bits")
                n2933 = VISA Close(VISA resource name=w3934, error in (no error)=w3935) -> (error out=w3933:errorcluster)
                n2934 = local write "humid"("" ("humid")) -> ()
                n2935 = local write "Humidity Str Rec"("" ("Humidity Str Rec")) -> ()
                n2936 = call <vilib>:"Clear Errors.vi"("error in (no error)"=w3933) -> ("error out"=w3932:errorcluster)  [unwired: 5 in, 1 out]
                n2937 = local read "Com Port 3"() -> (w3931:refnum<visa-resource-name>)
                n2938 = call-poly "VISA Configure Serial Port"("VISA resource name"=w3931, "timeout (10sec)"=u32 1000, "termination char\n(0xA = '\\n' = LF)"=u8 10 ("termination char\n(0xA = '\\n' = LF)"), "Enable Termination\nChar (T)"=FALSE ("Enable Termination Char (T)"), "baud rate (9600)"="Humidity BaudRate", "data bits (8)"=u16 8 ("data bits"), "parity (0:none)"=w3938, "error in (no error)"=w3932, "stop bits (10: 1 bit)"=w3941, "flow control (0:none)"=w3942) -> ("VISA resource name out"=w3937:refnum<visa-resource-name>, "error out"=w3928:errorcluster)  [unwired: 4 in]
              }
            }
            n2939 = Compound Arithmetic op=AND(w3833, w3832, w3834) -> (w3831:bool)
            n2940 = case shown="True" w3831 {
              tunnel: w3830 -> [_ _]
              tunnel: w3839 -> [_ w3869]
              frame False {
              }
              frame True {
                w3867 = " " ("regular expression")
                n2941 = Match Pattern(string=w3869, regular expression=" ") -> (after substring=w3871:string)  [unwired: 1 in, 3 out]
                n2942 = Match Pattern(string=w3871, regular expression=w3867) -> (before substring=→"humid":string, after substring=w3868:string)  [unwired: 1 in, 2 out]
                n2943 = Match Pattern(string=w3868, regular expression=w3867) -> (before substring=→"temp_@Rh sensor":string)  [unwired: 1 in, 3 out]
              }
            }
            n2944 = local read "Quit"() -> (w3820:bool)
          }
          n2945 = VISA Close(VISA resource name=w3816, error in (no error)=w3817) -> (error out=w3813:errorcluster)
          n2946 = call <vilib>:"Clear Errors.vi"("error in (no error)"=w3813) -> ()  [unwired: 5 in, 2 out]
        }
        frame Enabled {
        }
      }
    }
    frame Enabled {
    }
  }
  n2947 = while {
    tunnel: [w3950] -> _
    i -> [w3950]
    stop <- w3945 stop-if-true
    # "Langauage selection"
    n2948 = property on="FF Calibration g" class="WFGraph (strict)"("Plot Area:Colors:FG Color"=u32 0) -> ()  [unwired: 2 in, 2 out]
    n2949 = Equal?(x="Lan flag", y=22.0) -> ()  [unwired: 1 out]
    n2950 = disable-structure shown="Disabled" {
      frame Disabled {
        n2951 = stacked-sequence {
          frame #0 {
            n2952 = case shown="\"Russian\"" "Language Selection" {
              tunnel: [0 1] -> w3952
              frame "English", Default {
              }
              frame "Russian" {
              }
            }
            n2953 = for {
              N: 130 -> [_]
              tunnel: "Table" -> [w3961]
              tunnel: w3952 -> [w3960]
              i -> [w3959]
              n2954 = Index Array(array=w3961, index (row)=w3959, index (col)=w3960) -> (element=w3958:string)
              n2955 = case shown="4" w3959 {
                tunnel: w3958 -> [w3962 w3963 _ w3964 w3965 w3966 w3967 w3968 w3969 w3970 w3971 w3972 w3973 w3974 w3975 w3976 w3977 w3978 w3979 w3980 w3981 w3982 w3983 w3984 w3985 w3986 w3987 w3988 w3989 _ _ w3990 w3991 w3992 w3993 w3994 w3995 w4004 w4011 w4018 w4025 w4029 w4032 w4035 w4037 w4039 w4040 w4041 w4042 w4043 w4044 w4045 w4046 w4047 w4048 w4049 w4050 w4051 w4052 w4053 w4054 w4055 w4056 w4057 w4058 w4059 w4060 w4061 w4062 w4063 w4064 w4065 w4066 w4067 w4068 w4069 w4070 w4071 w4072 w4073 w4074 w4075 w4076 w4077 w4078 w4079 w4080 w4081 w4082 w4083 w4084 w4085 w4086 w4087 w4088 w4089 w4090 w4091 w4092 w4093 w4094 w4095 w4096 w4097 w4098 _ w4099 w4100 w4101 w4102 w4103 w4104 w4105 w4106 w4107 w4108 w4109 w4110 w4111 _ w4112 w4113 w4114 w4115 w4116 w4117 _]
                frame 0 {
                  n2956 = local write "S"(w3962) -> ()
                }
                frame 1 {
                  n2957 = local write "S 2"(w3963) -> ()
                }
                frame 2 {
                }
                frame 3 {
                  n2958 = local write "S 4"(w3964) -> ()
                }
                frame 4 {
                  n2959 = property on="FILE" class="Str"("Caption.Text"=w3965) -> ()  [unwired: 2 in, 2 out]
                }
                frame 5 {
                  n2960 = property on="Fuel Discription :" class="Str"("Caption.Text"=w3966) -> ()  [unwired: 2 in, 2 out]
                }
                frame 6 {
                  n2961 = property on="Remarks :" class="Str"("Caption.Text"=w3967) -> ()  [unwired: 2 in, 2 out]
                }
                frame 7 {
                  n2962 = property on="Save & Continue" class="Bool (strict)"("Boolean Text.Text"=w3968) -> ()  [unwired: 2 in, 2 out]
                }
                frame 8 {
                }
                frame 9 {
                  n2963 = property on="Set Hz" class="DigNum (strict)"("Caption.Text"=w3970) -> ()  [unwired: 2 in, 2 out]
                }
                frame 10 {
                  "String 3" <- w3971
                }
                frame 11 {
                  n2964 = property on="NORMAL LOAD" class="DigNum (strict)"("Caption.Text"=w3972) -> ()  [unwired: 2 in, 2 out]
                }
                frame 12 {
                  "String 5" <- w3973
                }
                frame 13 {
                  n2965 = property on="Set Temp" class="DigNum (strict)"("Caption.Text"=w3974) -> ()  [unwired: 2 in, 2 out]
                }
                frame 14 {
                  n2966 = local write "S 15"(w3975) -> ()
                }
                frame 15 {
                  n2967 = property on="Set Rh" class="DigNum (strict)"("Caption.Text"=w3976) -> ()  [unwired: 2 in, 2 out]
                }
                frame 16 {
                  "String 13" <- w3977
                  "String 26" <- w3977
                }
                frame 17 {
                  n2968 = local write "S 18"(w3978) -> ()
                }
                frame 18 {
                  "String 17" <- w3979
                }
                frame 19 {
                  n2969 = property on="test time" class="DigNum (strict)"("Caption.Text"=w3980) -> ()  [unwired: 2 in, 2 out]
                }
                frame 20 {
                  "String 18" <- w3981
                  "String 22" <- w3981
                }
                frame 21 {
                  n2970 = property on="Elapsed time" class="DigNum (strict)"("Caption.Text"=w3982) -> ()  [unwired: 2 in, 2 out]
                }
                frame 22 {
                  n2971 = property on="Samplingtime 2" class="DigNum (strict)"("Caption.Text"=w3983) -> ()  [unwired: 2 in, 2 out]
                }
                frame 23 {
                  "String 21" <- w3984
                }
                frame 24 {
                  n2972 = property on="Countdown" class="DigNum (strict)"("Caption.Text"=w3985) -> ()  [unwired: 2 in, 2 out]
                }
                frame 25 {
                  n2973 = property on="Countdown 2" class="DigNum (strict)"("Caption.Text"=w3986) -> ()  [unwired: 2 in, 2 out]
                }
                frame 26 {
                  n2974 = property on="Engage" class="Bool (strict)"("Boolean Text.Text"=w3987) -> ()  [unwired: 2 in, 2 out]
                }
                frame 27 {
                  n2975 = property on="Boolean  4" class="Bool (strict)"("Boolean Text.Text"=w3988) -> ()  [unwired: 2 in, 2 out]
                }
                frame 28 {
                  n2976 = property on="Test \nStatus" class="Bool (strict)"("Boolean Text.Text"=w3989) -> ()  [unwired: 2 in, 2 out]
                }
                frame 29 {
                }
                frame 30 {
                }
                frame 31 {
                  n2977 = property on="FF Calibration g" class="WFGraph (strict)"("X Scale.Name Label.Text"=w3990) -> ()  [unwired: 2 in, 2 out]
                }
                frame 32 {
                  n2978 = property on="RSTCOF" class="Bool"("Boolean Text.Text"=w3991) -> ()  [unwired: 2 in, 2 out]
                  n2979 = property on="RST FF" class="Bool"("Boolean Text.Text"=w3991) -> ()  [unwired: 2 in, 2 out]
                  n2980 = property on="RST TEMP" class="Bool"("Boolean Text.Text"=w3991) -> ()  [unwired: 2 in, 2 out]
                  n2981 = property on="RSTV1 3" class="Bool"("Boolean Text.Text"=w3991) -> ()  [unwired: 2 in, 2 out]
                  n2982 = property on="rstv2" class="Bool"("Boolean Text.Text"=w3991) -> ()  [unwired: 2 in, 2 out]
                  n2983 = property on="RSTV1 2" class="Bool"("Boolean Text.Text"=w3991) -> ()  [unwired: 2 in, 2 out]
                  n2984 = property on="RST CP" class="Bool"("Boolean Text.Text"=w3991) -> ()  [unwired: 2 in, 2 out]
                }
                frame 33 {
                  "S 61" <- w3992
                }
                frame 34 {
                  "String 23" <- w3993
                }
                frame 35 {
                  n2985 = property on="Rh Before" class="DigNum (strict)"("Caption.Text"=w3994) -> ()  [unwired: 2 in, 2 out]
                }
                frame 36 {
                  n2986 = Match Pattern(string=w3995, regular expression=",") -> (before substring=→"bs":string, after substring=→"as":string)  [unwired: 1 in, 2 out]
                  n2987 = property on="Rh After" class="DigNum (strict)"("Caption.Text"=w3995) -> ()  [unwired: 2 in, 2 out]
                }
                frame 37 {
                  n2988 = Match Pattern(string=w4004, regular expression=",") -> (before substring=w4003:string, after substring=w4002:string)  [unwired: 1 in, 2 out]
                  "bs" <- w4003
                  "as" <- w4002
                  n2989 = Concatenate Strings(w4003, w4002) -> (w3999:string)
                  n2990 = property on="Humidity before test 2" class="DigNum (strict)"("Caption.Text"=w3999) -> ()  [unwired: 2 in, 2 out]
                  n2991 = property on="Humidity before test" class="DigNum (strict)"("Caption.Text"=w3999) -> ()  [unwired: 2 in, 2 out]
                  n2992 = Concatenate Strings(w3999, "=" ("string")) -> (w4000:string)
                  n2993 = local write "S 38"(w4000) -> ()
                }
                frame 38 {
                  n2994 = Match Pattern(string=w4011, regular expression=",") -> (before substring=w4010:string, after substring=w4009:string)  [unwired: 1 in, 2 out]
                  "bs" <- w4010
                  "as" <- w4009
                  n2995 = Concatenate Strings(w4010, w4009) -> (w4006:string)
                  n2996 = property on="Humidity after test 2" class="DigNum (strict)"("Caption.Text"=w4006) -> ()  [unwired: 2 in, 2 out]
                  n2997 = Concatenate Strings(w4006, "=" ("string")) -> (w4008:string)
                  n2998 = property on="Humidity after test" class="DigNum (strict)"("Caption.Text"=w4006) -> ()  [unwired: 2 in, 2 out]
                  n2999 = local write "S 39"(w4008) -> ()
                }
                frame 39 {
                  n3000 = Match Pattern(string=w4018, regular expression=",") -> (before substring=w4017:string, after substring=w4016:string)  [unwired: 1 in, 2 out]
                  "bs" <- w4017
                  "as" <- w4016
                  n3001 = Concatenate Strings(w4017, w4016) -> (w4013:string)
                  n3002 = property on="Temperature before test 2" class="DigNum (strict)"("Caption.Text"=w4013) -> ()  [unwired: 2 in, 2 out]
                  n3003 = property on="Temperature before test" class="DigNum (strict)"("Caption.Text"=w4013) -> ()  [unwired: 2 in, 2 out]
                  n3004 = Concatenate Strings(w4013, "=" ("string")) -> (→"String 34":string)
                }
                frame 40 {
                  n3005 = Match Pattern(string=w4025, regular expression=",") -> (before substring=w4024:string, after substring=w4023:string)  [unwired: 1 in, 2 out]
                  "bs" <- w4024
                  "as" <- w4023
                  n3006 = Concatenate Strings(w4024, w4023) -> (w4020:string)
                  n3007 = property on="Temperature after test 2" class="DigNum (strict)"("Caption.Text"=w4020) -> ()  [unwired: 2 in, 2 out]
                  n3008 = Concatenate Strings(w4020, "=" ("string")) -> (→"String 35":string)
                  n3009 = property on="Temperature after test" class="DigNum (strict)"("Caption.Text"=w4020) -> ()  [unwired: 2 in, 2 out]
                }
                frame 41 {
                  n3010 = property on="AVP" class="DigNum (strict)"("Caption.Text"=w4029) -> ()  [unwired: 2 in, 2 out]
                  n3011 = property on="AVP 2" class="DigNum (strict)"("Caption.Text"=w4029) -> ()  [unwired: 2 in, 2 out]
                  n3012 = Concatenate Strings(w4029, "=" ("string")) -> (→"String 36":string)
                }
                frame 42 {
                  n3013 = property on="MWSD" class="DigNum (strict)"("Caption.Text"=w4032) -> ()  [unwired: 2 in, 2 out]
                  n3014 = property on="MWSD 2" class="DigNum (strict)"("Caption.Text"=w4032) -> ()  [unwired: 2 in, 2 out]
                  n3015 = Concatenate Strings(w4032, "=" ("string")) -> (→"String 37":string)
                }
                frame 43 {
                  n3016 = property on="HCF 2" class="DigNum (strict)"("Caption.Text"=w4035) -> ()  [unwired: 2 in, 2 out]
                  n3017 = property on="HCF" class="DigNum (strict)"("Caption.Text"=w4035) -> ()  [unwired: 2 in, 2 out]
                  n3018 = Concatenate Strings(w4035, "=" ("string")) -> (→"String 38":string)
                }
                frame 44 {
                  n3019 = Concatenate Strings(w4037, "=" ("string")) -> (→"String 39":string)
                  n3020 = property on="WS1.4 2" class="DigNum (strict)"("Caption.Text"=w4037) -> ()  [unwired: 2 in, 2 out]
                  n3021 = property on="WS1.4" class="DigNum (strict)"("Caption.Text"=w4037) -> ()  [unwired: 2 in, 2 out]
                }
                frame 45 {
                  n3022 = property on="Save Results" class="Bool (strict)"("Boolean Text.Text"=w4039) -> ()  [unwired: 2 in, 2 out]
                }
                frame 46 {
                  n3023 = local write "S 47"(w4040) -> ()
                }
                frame 47 {
                  n3024 = local write "S 48"(w4041) -> ()
                }
                frame 48 {
                  n3025 = local write "S 49"(w4042) -> ()
                }
                frame 49 {
                  n3026 = local write "S 50"(w4043) -> ()
                }
                frame 50 {
                  n3027 = local write "S 51"(w4044) -> ()
                }
                frame 51 {
                  n3028 = local write "S 52"(w4045) -> ()
                }
                frame 52 {
                  n3029 = local write "S 53"(w4046) -> ()
                }
                frame 53 {
                  n3030 = local write "S 54"(w4047) -> ()
                }
                frame 54 {
                  n3031 = local write "S 55"(w4048) -> ()
                }
                frame 55 {
                  n3032 = local write "S 56"(w4049) -> ()
                }
                frame 56 {
                  n3033 = local write "S 57"(w4050) -> ()
                }
                frame 57 {
                  n3034 = local write "S 58"(w4051) -> ()
                }
                frame 58 {
                  n3035 = local write "S 59"(w4052) -> ()
                }
                frame 59 {
                  n3036 = local write "S 60"(w4053) -> ()
                }
                frame 60 {
                  n3037 = local write "S 62"(w4054) -> ()
                }
                frame 61 {
                  n3038 = local write "S 63"(w4055) -> ()
                }
                frame 62 {
                  n3039 = local write "S 64"(w4056) -> ()
                }
                frame 63 {
                  n3040 = local write "S 65"(w4057) -> ()
                }
                frame 64 {
                  n3041 = local write "S 66"(w4058) -> ()
                }
                frame 65 {
                  n3042 = local write "S 67"(w4059) -> ()
                }
                frame 66 {
                  n3043 = local write "S 68"(w4060) -> ()
                }
                frame 67 {
                  n3044 = local write "S 69"(w4061) -> ()
                }
                frame 68 {
                  n3045 = local write "S 70"(w4062) -> ()
                }
                frame 69 {
                  n3046 = local write "S 71"(w4063) -> ()
                }
                frame 70 {
                  n3047 = local write "S 72"(w4064) -> ()
                }
                frame 71 {
                  n3048 = local write "S 73"(w4065) -> ()
                }
                frame 72 {
                  n3049 = local write "S 74"(w4066) -> ()
                }
                frame 73 {
                  n3050 = local write "S 75"(w4067) -> ()
                }
                frame 74 {
                  n3051 = local write "S 76"(w4068) -> ()
                }
                frame 75 {
                  n3052 = local write "S 77"(w4069) -> ()
                }
                frame 76 {
                  n3053 = local write "S 78"(w4070) -> ()
                }
                frame 77 {
                  n3054 = local write "S 79"(w4071) -> ()
                }
                frame 79 {
                  n3055 = property on="Sample Temperature ( °C )" class="XYGraph (strict)"("Y Scale.Name Label.Text"=w4072) -> ()  [unwired: 2 in, 2 out]
                }
                frame 80 {
                  n3056 = local write "S 81"(w4073) -> ()
                  n3057 = property on="Humidity ( %RH )" class="XYGraph (strict)"("Y Scale.Name Label.Text"=w4073) -> ()  [unwired: 2 in, 2 out]
                }
                frame 78 {
                  n3058 = property on="Air Temperature  ( °C )" class="XYGraph (strict)"("X Scale.Name Label.Text"=w4074) -> ()  [unwired: 2 in, 2 out]
                  n3059 = property on="Humidity ( %RH )" class="XYGraph (strict)"("X Scale.Name Label.Text"=w4074) -> ()  [unwired: 2 in, 2 out]
                  n3060 = property on="Sample Temperature ( °C )" class="XYGraph (strict)"("X Scale.Name Label.Text"=w4074) -> ()  [unwired: 2 in, 2 out]
                  n3061 = property on="Coefficient Of Friction" class="XYGraph (strict)"("X Scale.Name Label.Text"=w4074) -> ()  [unwired: 2 in, 2 out]
                }
